vi "Poisson PF.vi"(10 "lambda":dbl=1.0, 11 "x":i32=1) -> (0 "error":i32, 3 "prob(x)":dbl=0.36787944117144233)   [LabVIEW 2024, in "NI_Gmath.lvlib"]
doc: "<p>Computes the discrete <a href=\"nihelplauncher://docs/csh?context=lvcore_gmath_probability_distributions\">probability function</a> (PF), or the probability that the random variate <em>X</em>, where <em>X</em> describes the selected distribution type, takes on the value <strong>n</strong>. You must <a href=\"nihelplauncher://docs/csh?context=lvcore_lvhowto_selectingdefaultinstpolyvi\">manually select the polymorphic instance</a> to use.</p>"
uses:
  NI_Gmath.lvlib
panel:
  # "Poisson PF"
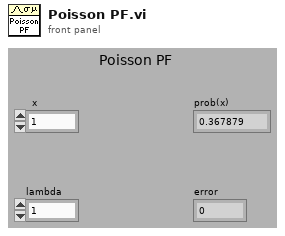
[diagram p1: front panel]
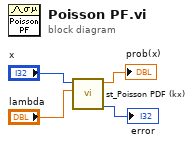
[diagram p0: block diagram]
diagram:
  n1 = call "st_Poisson PDF (kx).vi"("a"="lambda", "x"="x") -> ("error"=→"error":i32, "pdf(x)"=→"prob(x)":dbl)  [unwired: 8 in]
